vi "FaceTracking.vi"() -> ()   [LabVIEW 2019]
doc: "This example demonstrates the Traditional MeanShift algorithm to track an object in the image."
panel:
  out "Image 2":T1(plugin-control)
  out "size(s)":i32
  out "Image":T1(plugin-control)
  in  "Stop":bool
  in  "Delay (s.)":dbl(slide) scale=0.0..2.0
  # "Overview: Demonstrate the Traditional MeanShift algorithm to track an object in the image.\nRequirements: LabVIEW Full Development System and Vision Development Module.\nInstructions: Run the VI."
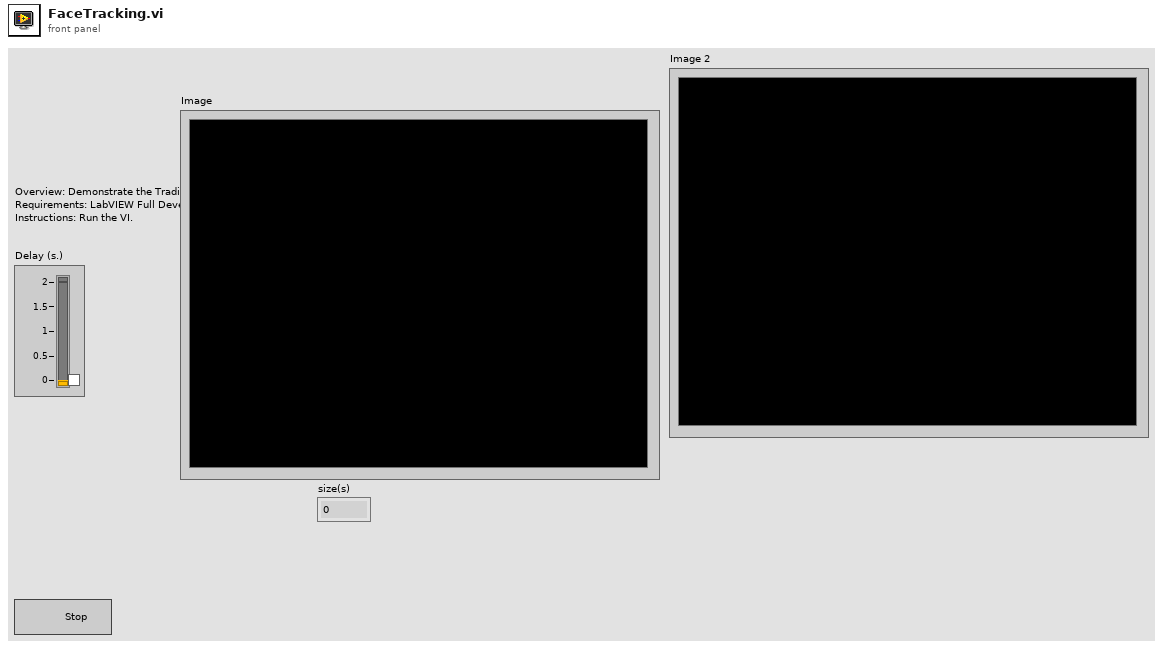
[diagram p1: front panel]
types:
  T1 = typedef "IMAQ Image.ctl" = refnum<image>
  T2 = cluster{"Number of Histogram Bins":i32, "Blending Parameter (%)":dbl, "Maximum Iterations":i32}
  T3 = typedef "Image Type" = u32
  T4 = typedef "IMAQ Object Tracking Session.ctl" = refnum<k20>
  T5 = typedef "IMAQ AVI2 Refnum.ctl" = refnum<k20>
  T6 = cluster{"Label":string, "Score":i32, "Angle":dbl, "Location":cluster{"X":dbl, "Y":dbl}, "Bounding Box":cluster{"X":dbl, "Y":dbl}[], "Object Found?":bool}[]
  T7 = typedef "IMAQ Rectangle" = cluster{"Left":i32, "Top":i32, "Right":i32, "Bottom":i32, "Rotation":dbl}
  T8 = typedef "ROI Descriptor" = cluster{"Global Rectangle":i32[], "Contours":cluster{"ID":enum32{"External", "Internal"}, "Type":u32, "Coordinates":i32[]}[]}
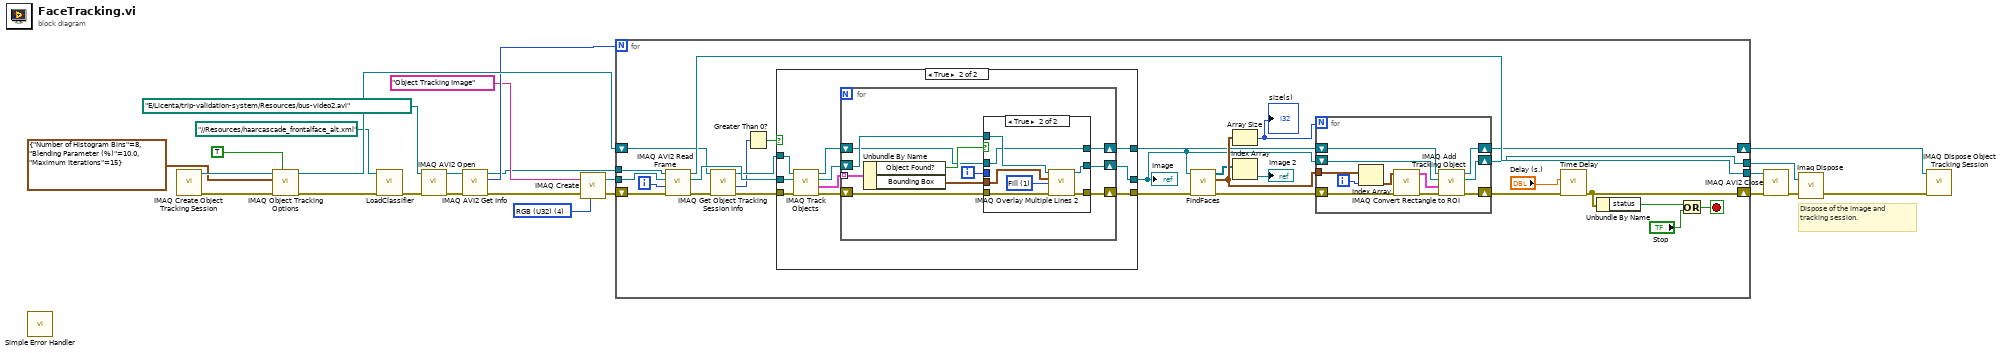
[diagram p0: block diagram]
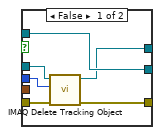
[diagram p3: hidden frame]
diagram:
  w12 = T3 4 items=["Grayscale (U8)", "Grayscale (I16)", "Grayscale (SGL)", "Complex (CSG)", "RGB (U32)", "HSL (U32)", "RGB (U64)", "Grayscale (U16)"] ("Image Type")
  # "Dispose of the image and tracking session."
  n1 = call <vilib>:"Simple Error Handler.vi"() -> ()  [unwired: 2 in, 8 out]
  n2 = call "IMAQ Create Object Tracking Session"() -> ("error out"=w18:errorcluster, "Object Tracking Session"=w21:T4)  [unwired: 1 in, 9 out]
  n3 = call-poly "IMAQ Object Tracking Options"("Get/Set (Get)"=TRUE, "error in (no error)"=w18, "Mean Shift Options in"=T2 {"Number of Histogram Bins"=8, "Blending Parameter (%)"=10.0, "Maximum Iterations"=15}, "Object Tracking Session In"=w21) -> ("error out"=w3:errorcluster, "Object Tracking Session Out"=w20:T4)  [unwired: 5 in, 1 out]
  n4 = call "LoadClassifier.vi"("error in (no error)"=w3, "faceCascadePath"=path "../../Resources/haarcascade_frontalface_alt.xml" ("Face Cascade Path")) -> ("error out"=w2:errorcluster)  [unwired: 9 in]
  n5 = call "IMAQ AVI2 Open"("error in (no error)"=w2, "AVI File Path"=path "E:/Licenta/trip-validation-system/Resources/bus-video2.avi") -> ("error out"=w16:errorcluster, "AVI Refnum"=w17:T5)  [unwired: 8 in]
  n6 = call "IMAQ AVI2 Get Info"("error in (no error)"=w16, "AVI Refnum"=w17) -> ("error out"=w13:errorcluster, "Number of Frames"=w15:u32, "AVI Refnum (duplicate)"=w11:T5)  [unwired: 5 in, 2 out]
  n7 = call "IMAQ Create"("Image Name"="Object Tracking Image", "Image Type"=w12, "error in (no error)"=w13) -> ("New Image"=w10:T1, "error out"=w9:errorcluster)  [unwired: 2 in]
  n8 = for {
    N: w15 -> [_]
    tunnel: [w28] -> w24
    shift-right: [w37] -> w23
    shift-left: w20 -> [w34]
    tunnel: w11 -> [w50]
    tunnel: w10 -> [w49]
    shift-right: [w44] -> w7
    shift-left: w9 -> [w45]
    tunnel: [w43] -> w8
    i -> [w48]
    stop <- w46 stop-if-true
    n9 = call "IMAQ AVI2 Read Frame"("error in (no error)"=w45, "Frame Number"=w48, "Image"=w49, "AVI Refnum"=w50) -> ("error out"=w30:errorcluster, "Image Out"=w42:T1, "AVI Refnum (duplicate)"=w43:T5)  [unwired: 5 in]
    n10 = call "IMAQ Get Object Tracking Session Info"("error in (no error)"=w30, "Object Tracking Session In"=w34) -> ("error out"=w29:errorcluster, "Number of Objects"=w31:i32, "Object Tracking Session Out"=w33:T4)  [unwired: 6 in, 1 out]
    n11 = Greater Than 0?(x=w31) -> (x > 0?=w32:bool)
    n12 = case shown="True" w32 {
      tunnel: w42 -> [w54 w63]
      tunnel: w33 -> [w55 w62]
      tunnel: w29 -> [w53 w61]
      tunnel: [w53 w60] -> w41
      tunnel: [w54 w59] -> w27
      tunnel: [w55 w56] -> w38
      frame False {
      }
      frame True {
        n13 = call "IMAQ Track Objects"("error in (no error)"=w61, "Image"=w63, "Object Tracking Session In"=w62) -> ("error out"=w64:errorcluster, "Objects (pixel)"=w58:T6, "Image (duplicate)"=w65:T1, "Object Tracking Session Out"=w57:T4)  [unwired: 1 in, 4 out]
        n14 = for {
          shift-right: [w69] -> w59
          shift-left: w65 -> [w70]
          shift-right: [w72] -> w60
          shift-left: w64 -> [w74]
          tunnel: w58 -> [w71] mode=indexing
          shift-right: [w66] -> w56
          shift-left: w57 -> [w67]
          i -> [w68]
          n15 = Unbundle By Name(w71) -> ("Object Found?"=w73:bool, "Bounding Box"=w75:cluster{"X":dbl, "Y":dbl}[])
          n16 = case shown="True" w73 {
            tunnel: w70 -> [w81 w88]
            tunnel: [w81 w87] -> w69
            tunnel: w75 -> [_ w86]
            tunnel: w74 -> [w79 w85]
            tunnel: [w78 w84] -> w72
            tunnel: w68 -> [w80 _]
            tunnel: w67 -> [w77 w82]
            tunnel: [w76 w82] -> w66
            frame False {
              n17 = call "IMAQ Delete Tracking Object"("error in (no error)"=w79, "Object Index"=w80, "Object Tracking Session In"=w77) -> ("error out"=w78:errorcluster, "Object Tracking Session Out"=w76:T4)  [unwired: 7 in]
            }
            frame True {
              w83 = u32 1 items=["Frame", "Fill"] ("Drawing Mode (Frame)")
              n18 = call "IMAQ Overlay Multiple Lines 2"("Image"=w88, "Line End Points"=w86, "Drawing Mode (Frame)"=w83, "error in (no error)"=w85) -> ("Image Out"=w87:T1, "error out"=w84:errorcluster)  [unwired: 4 in, 6 out]
            }
          }
        }
      }
    }
    "Image" <- w27
    n19 = call "FindFaces.vi"("error in"=w41, "Image In"=w27) -> ("error out"=w36:errorcluster, "Faces"=w39:T7[], "Array"=w26:T1[])  [unwired: 7 in]
    n20 = Array Size(array=w39) -> (size(s)=w40:i32)
    "size(s)" <- w40
    n21 = Index Array(array=w26) -> (element=→"Image 2":T1)  [unwired: 1 in]
    n22 = for {
      N: w40 -> [_]
      tunnel: w39 -> [w92]
      shift-right: [w97] -> w37
      shift-left: w38 -> [w98]
      shift-right: [w93] -> w35
      shift-left: w36 -> [w94]
      shift-right: [w89] -> w28
      shift-left: w27 -> [w99]
      i -> [w90]
      n23 = Index Array(array=w92, index=w90) -> (element=w91:T7)
      n24 = call "IMAQ Convert Rectangle to ROI"("error in (no error)"=w94, "Rectangle"=w91) -> ("error out"=w95:errorcluster, "ROI Descriptor"=w96:T8)  [unwired: 7 in]
      n25 = call "IMAQ Add Tracking Object"("error in (no error)"=w95, "ROI Descriptor"=w96, "Image"=w99, "Object Tracking Session In"=w98) -> ("error out"=w93:errorcluster, "Image (duplicate)"=w89:T1, "Object Tracking Session Out"=w97:T4)  [unwired: 1 in, 4 out]
    }
    n26 = call "Time Delay"("error in (no error)"=w35, "Delay Time (s)"="Delay (s.)") -> ("error out"=w44:errorcluster)  [unwired: 9 in]
    n27 = Unbundle By Name(w44) -> ("status"=w52:bool)
    n28 = Or(x=w52, y="Stop") -> (x .or. y?=w46:bool)
  }
  n29 = call "IMAQ AVI2 Close"("error in (no error)"=w7, "AVI Refnum"=w8) -> ("error out"=w6:errorcluster)  [unwired: 9 in]
  n30 = call "Imaq Dispose"("Image"=w24, "error in (no error)"=w6) -> ("error out"=w22:errorcluster)  [unwired: 1 in, 3 out]
  n31 = call "IMAQ Dispose Object Tracking Session"("error in (no error)"=w22, "Object Tracking Session"=w23) -> ()  [unwired: 10 out]
